vi "MakeDataFileForMultiplot.vi"(4 "Y Axis Name":string, 5 "Plot Array":cluster{"Angle":dbl[], "Radius":dbl[]}[](array[cluster]), 6 "X Axis Name":string, 7 "Path":path, 8 "Error Bar Cluster":cluster{string[]}[](array[cluster]), 9 "Transpose":bool, 10 "Plot Summary":string[][](array[string]), 11 "Legend":string[](array[string])) -> ()   [LabVIEW 2014]
uses:
  Results_plotter_Global.vi
panel:
  out "datLoops":i32
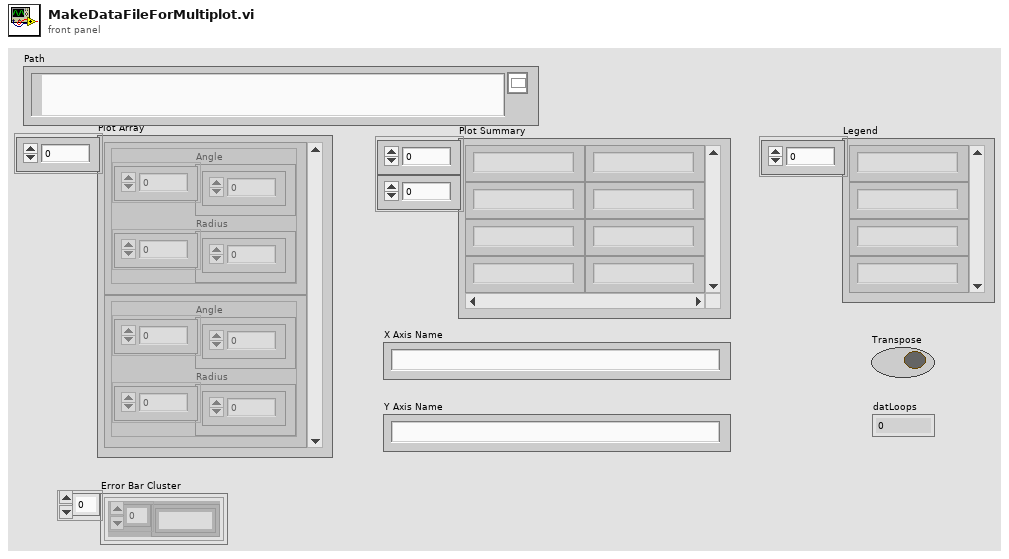
[diagram p1: front panel]
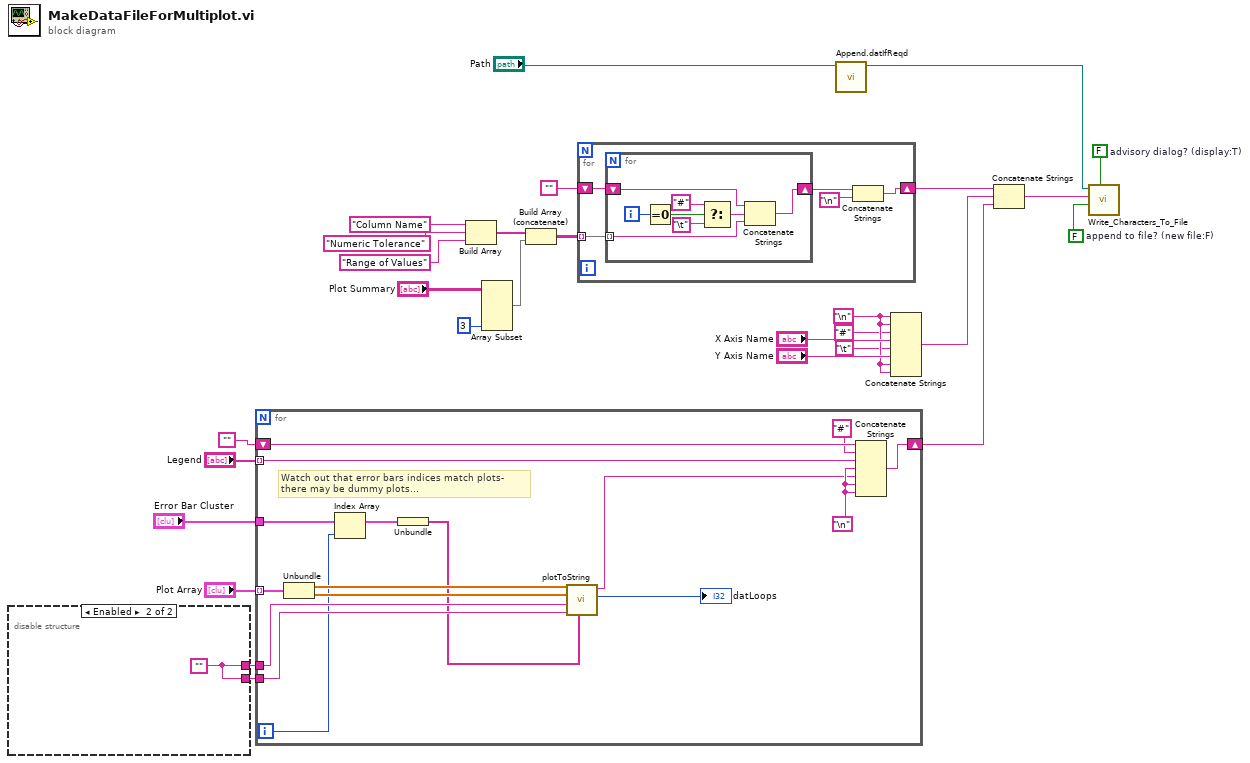
[diagram p0: block diagram]
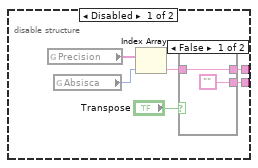
[diagram p2: hidden frame]
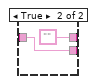
[diagram p3: hidden frame]
diagram:
  w8 = FALSE  # advisory dialog? (display:T)
  w7 = FALSE  # append to file? (new file:F)
  w17 = "\n"
  n1 = disable-structure shown="Enabled" {
    disable-tunnel: [w30 w39] -> w11
    disable-tunnel: [w29 w39] -> w10
    frame Disabled {
      n2 = global read "Results_plotter_Global.vi" "Precision"() -> (w31:string[])
      n3 = global read "Results_plotter_Global.vi" "Absisca"() -> (w32:i32)
      n4 = Index Array(array=w31, index=w32) -> (element=w33:string)
      n5 = case shown="False" "Transpose" {
        tunnel: ["" w38] -> w29
        tunnel: w33 -> [w35 w38]
        tunnel: [w35 ""] -> w30
        frame False {
        }
        frame True {
        }
      }
    }
    frame Enabled {
      w39 = ""
    }
  }
  n6 = for {
    tunnel: "Plot Array" -> [w55] mode=indexing
    shift-right: [w54] -> w3
    shift-left: "" -> [w49]
    tunnel: "Legend" -> [w47] mode=indexing
    tunnel: w11 -> [w46]
    tunnel: w10 -> [w44]
    tunnel: "Error Bar Cluster" -> [w43]
    i -> [w40]
    w53 = "\n"
    # "Watch out that error bars indices match plots-\nthere may be dummy plots..."
    n7 = Unbundle(w55) -> ("Angle"=w50:dbl[], "Radius"=w51:dbl[])
    n8 = Index Array(array=w43, index=w40) -> (element=w41:cluster{string[]})
    n9 = Unbundle(w41) -> (w42:string[])
    n10 = call "plotToString.vi"("Error Bar values"=w42, "Precision2"=w44, "Precision1"=w46, "Column2"=w51, "Column1"=w50) -> ("nLoops"=→"datLoops":i32, "plotString"=w52:string)  [unwired: 5 in]
    n11 = Concatenate Strings(w49, "#", w47, w53, w52, w53, w53) -> (w54:string)
  }
  n12 = Build Array("Column Name", "Numeric Tolerance", "Range of Values") -> (w20:string[])
  n13 = Array Subset(array="Plot Summary", length (col)=3 ("length")) -> (w25:string[][])  [unwired: 3 in]
  n14 = Build Array (concatenate)(w20, w25) -> (w27:string[][])
  n15 = for {
    shift-right: [w59] -> w5
    shift-left: "" -> [w56]
    tunnel: w27 -> [w60] mode=indexing
    n16 = for {
      shift-right: [w61] -> w58
      shift-left: w56 -> [w68]
      tunnel: w60 -> [w62] mode=indexing
      i -> [w67]
      n17 = Equal To 0?(x=w67) -> (x = 0?=w66:bool)
      n18 = Select(t="#", s=w66, f="\t") -> (s? t:f=w63:string)
      n19 = Concatenate Strings(w68, w63, w62) -> (w61:string)
    }
    n20 = Concatenate Strings(w58, "\n") -> (w59:string)
  }
  n21 = call "Append.datIfReqd.vi"("Path"="Path") -> ("appended path"=w9:path)  [unwired: 10 in]
  n22 = Concatenate Strings(w17, w17, "#" ("string"), "X Axis Name", "\t", "Y Axis Name", w17, w17) -> (w4:string)
  n23 = Concatenate Strings(w5, w4, w3) -> (w6:string)
  n24 = call "Write_Characters_To_File.vi"("file path (dialog if empty)"=w9, "advisory dialog? (display:T)"=w8, "character string"=w6, "append to file? (new file:F)"=w7) -> ()  [unwired: 1 in, 4 out]
